vi "FlpLib Derivative 0.vi"(1 "dt":sgl, 7 "x":sgl format="%#_13g") -> (8 "dx":sgl format="%#_13g")   [LabVIEW 2017]
uses:
  <userlib>/_NI FLP Library/FPGA/outsideSCTL/FlpLib Subtract Shared Instance 0.vi
  <userlib>/_NI FLP Library/FPGA/outsideSCTL/FlpLib Multiply Shared Instance 0.vi
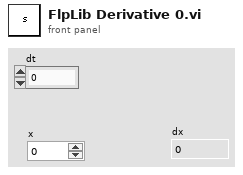
[diagram p1: front panel]
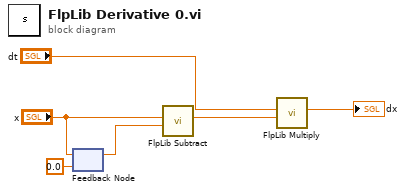
[diagram p0: block diagram]
diagram:
  n1 = feedback-in #1("x") -> ()
  n2 = feedback #1(sgl 0.0 ("x")) -> (w5:sgl)
  n3 = call-poly <userlib>:"FlpLib Subtract.vi"("y"=w5, "x"="x") -> ("x-y"=w4:sgl)  [unwired: 5 in]
  n4 = call-poly <userlib>:"FlpLib Multiply.vi"("y"=w4, "x"="dt") -> ("x*y"=→"dx":sgl)  [unwired: 5 in]
